vi "Event_Register.vi"(4 "error in (no error)":errorcluster, 7 "UsbDllWrap":refnum<k24>) -> (0 "error out":errorcluster, 1 "Event Callback Refnum":refnum<k27>, 2 "DeviceStateChangedEvent":refnum<user-event>, 3 "Event Registration Refnum":refnum<event-registration>)   [LabVIEW 2009]
uses:
  C:/Samples/LabVIEW/UseEventHandling/LabVIEW 2009/UsbDllWrap.dll
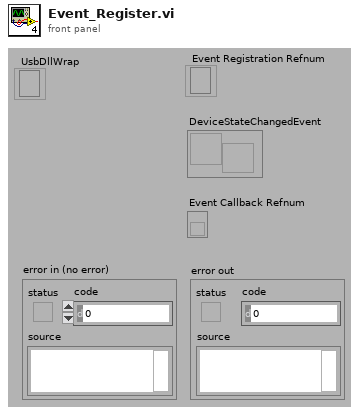
[diagram p1: front panel]
types:
  T1 = cluster{"Device Key":string, "Device State":refnum<k24>}
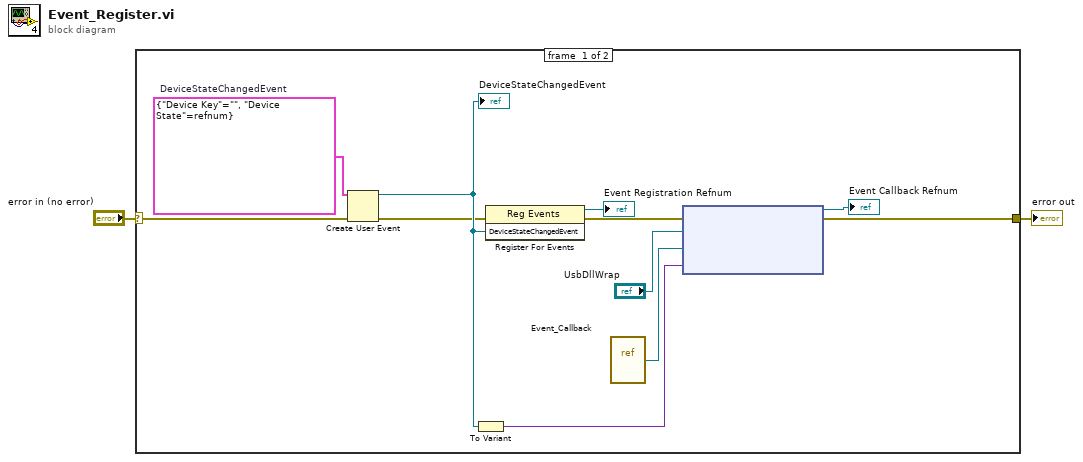
[diagram p0: block diagram]
diagram:
  n1 = case shown="No Error" "error in (no error)" {
    selector: "error in (no error)" -> [w13 w14]
    tunnel: [w10 w14] -> w2
    frame #0 {
      w12 = T1 {"Device Key"="", "Device State"=refnum}  # DeviceStateChangedEvent
      n2 = Create User Event(user event datatype=w12, error in=w13) -> (user event=w7:refnum<user-event>, error out=w5:errorcluster)
      "DeviceStateChangedEvent" <- w7
      n3 = To Variant(anything=w7) -> (Variant=w11:variant)
      n4 = register-events(error in=w5, w7) -> (reference out=→"Event Registration Refnum":refnum<event-registration>, error out=w6:errorcluster)  [unwired: 1 in]
      n5 = vi-ref "Event_Callback.vi"() -> ("vi reference"=w4:refnum<vi>)
      n6 = node(w6, "UsbDllWrap", w4, w11) -> (→"Event Callback Refnum":refnum<k27>, w10:errorcluster)  [unwired: 1 in]
    }
    frame #1 {
    }
  }
  "error out" <- w2
